vi "WaitMove.vi"(0 "Axis In":T1, 5 "Polling Interval in ms (20)":u32=20, 11 "error in (no error)":errorcluster) -> (4 "Axis Out":T1, 15 "error out":errorcluster)   [LabVIEW 2009]
doc: "Waits until axis is in position or an error occurs."
uses:
  typedefs/AxisSelect_Enum.ctl
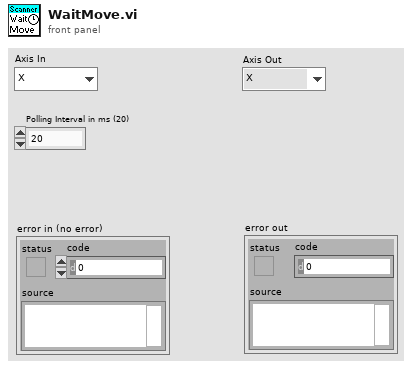
[diagram p1: front panel]
types:
  T1 = typedef "AxisSelect_Enum.ctl" = enum16{"X", "Y", "Z", "Axis Space"}
  T2 = typedef "DriveStatus_Cluster.ctl" = cluster{"In-position":bool, "Zero Speed":bool, "Enabled":bool, "Fault Disable":bool, "Ready":bool, "Start Index":bool, "Overtravel Exceeded":bool, "Up to Speed":bool, "Sequence Complete":bool}
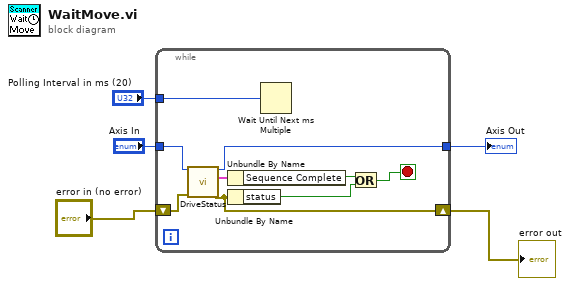
[diagram p0: block diagram]
diagram:
  n1 = while {
    tunnel: "Axis In" -> [w12]
    tunnel: "Polling Interval in ms (20)" -> [w13]
    tunnel: [w11] -> w3
    shift-right: [w7] -> w1
    shift-left: "error in (no error)" -> [w6]
    stop <- w14 stop-if-true
    n2 = call "DriveStatus.vi"("Axis In"=w12, "error in (no error)"=w6) -> ("Axis Out"=w11:T1, "Status"=w10:T2, "error out"=w7:errorcluster)  [unwired: 11 in]
    n3 = Unbundle By Name(w10) -> ("Sequence Complete"=w9:bool)
    n4 = Unbundle By Name(w7) -> ("status"=w8:bool)
    n5 = Wait Until Next ms Multiple(millisecond multiple=w13) -> ()  [unwired: 1 out]
    n6 = Or(x=w9, y=w8) -> (x .or. y?=w14:bool)
  }
  "Axis Out" <- w3
  "error out" <- w1
